vi "CRYSignal Path Table.vi"(11 "Calibration":T1[](array[typedef]) {"Sens Curve"."Z data" items=["dB", "Lin"]; "Sens Curve"."X data" items=["dB", "Lin"]; "Sens Curve"."Y data" items=["dB", "Lin"]; "Sens Curve"."Z dB ref" format="%.1f"; "Sens Curve"."Z axis" items=["Log", "Lin"]; "Sens Curve"."X dB ref" format="%.1f"; "Sens Curve"."X axis" items=["Log", "Lin"]; "Sens Curve"."Y axis" items=["Log", "Lin"]; "Sens Curve"."Y dB ref" format="%.1f"; "Sens Curve"."Curve"."z" format="%.2f"; "Sens Curve"."Curve"."y" format="%.2f"; "Sens Curve"."Curve"."x" format="%.2f"; "EQ Curve"."Z data" items=["dB", "Lin"]; "EQ Curve"."X data" items=["dB", "Lin"]; "EQ Curve"."Y data" items=["dB", "Lin"]; "EQ Curve"."Z dB ref" format="%.1f"; "EQ Curve"."Z axis" items=["Log", "Lin"]; "EQ Curve"."X dB ref" format="%.1f"; "EQ Curve"."X axis" items=["Log", "Lin"]; "EQ Curve"."Y axis" items=["Log", "Lin"]; "EQ Curve"."Y dB ref" format="%.1f"; "EQ Curve"."Curve"."z" format="%.2f"; "EQ Curve"."Curve"."y" format="%.2f"; "EQ Curve"."Curve"."x" format="%.2f"; "Corr Curve"."Z data" items=["dB", "Lin"]; "Corr Curve"."X data" items=["dB", "Lin"]; "Corr Curve"."Y data" items=["dB", "Lin"]; "Corr Curve"."Z dB ref" format="%.1f"; "Corr Curve"."Z axis" items=["Log", "Lin"]; "Corr Curve"."X dB ref" format="%.1f"; "Corr Curve"."X axis" items=["Log", "Lin"]; "Corr Curve"."Y axis" items=["Log", "Lin"]; "Corr Curve"."Y dB ref" format="%.1f"; "Corr Curve"."Curve"."z" format="%.2f"; "Corr Curve"."Curve"."y" format="%.2f"; "Corr Curve"."Curve"."x" format="%.2f"; "Calibration"."EQ Step size" items=["R10", "R20", "R40", "R80", "User"]; "Calibration"."Corr Step size" items=["R10", "R20", "R40", "R80", "User"]}) -> ()   [LabVIEW 2013]
uses:
  Typedef Control/CRYCalibration 2DCluster.ctl
  Typedef Control/CRYCalibration Cluster.ctl
  Typedef Control/CRYData Cluster.ctl
panel:
  out "OutputTable":string[][](table) caption="aaa"
  in  "OK":bool
  out "InputTable":string[][](table) caption="aaa"
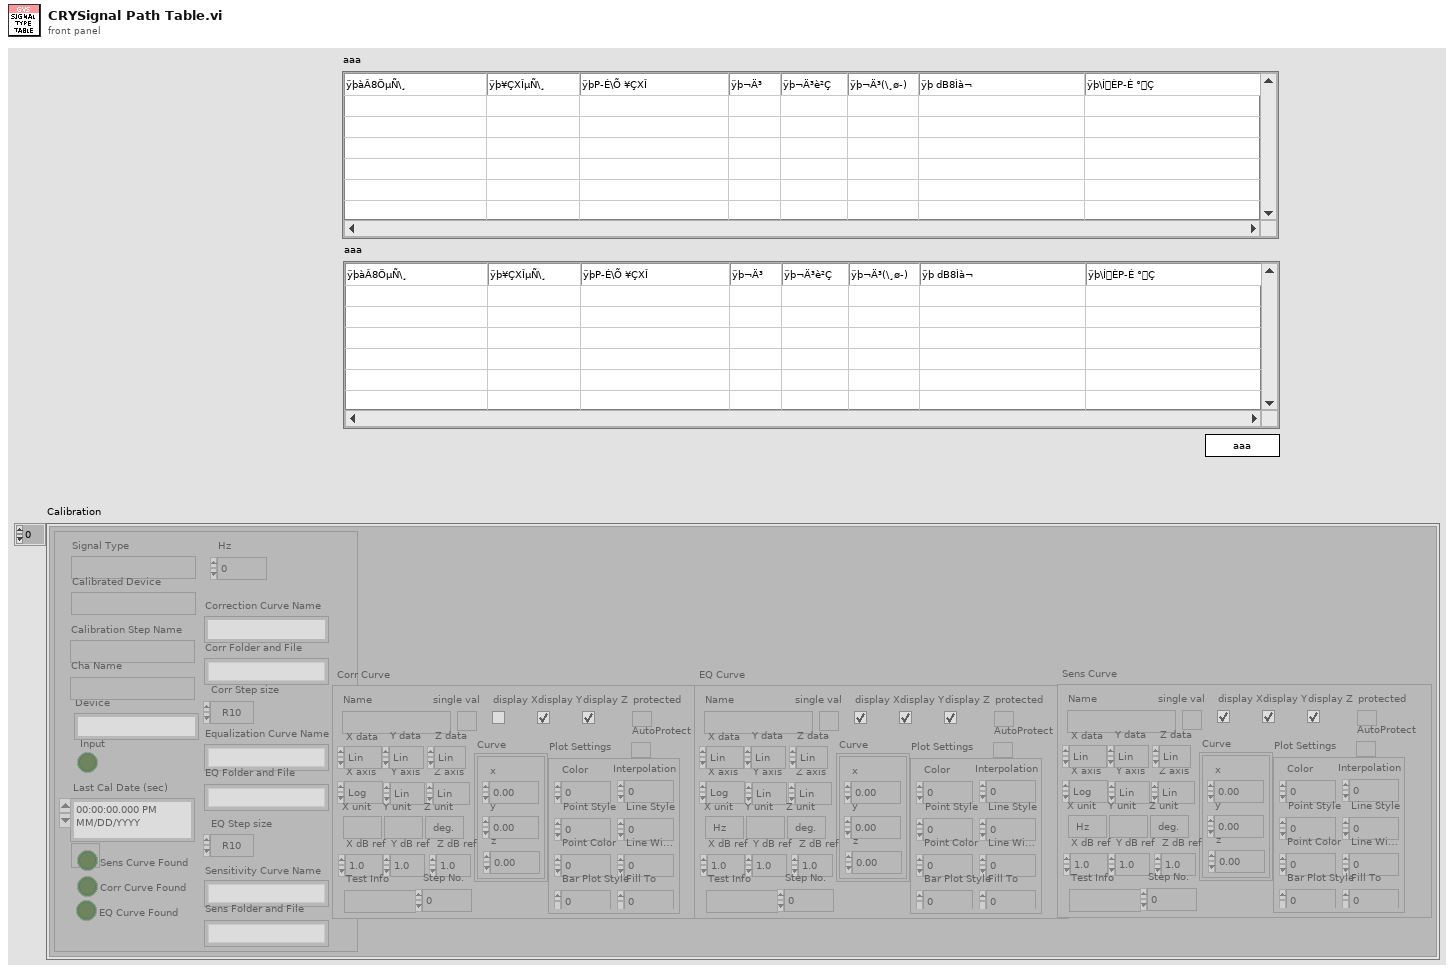
[diagram p1: front panel]
types:
  T1 = typedef "CRYCalibration 2DCluster.ctl" = cluster{"Calibration":T2, "Corr Curve":T3, "EQ Curve":T3, "Sens Curve":T3}
  T2 = typedef "CRYCalibration Cluster.ctl" = cluster{"Calibration Step Name":string, "Device":string, "Correction Curve Name":string, "Equalization Curve Name":string, "Sensitivity Curve Name":string, "Corr Folder and File":string, "EQ Folder and File":string, "Sens Folder and File":string, "Corr Step size":u16, "EQ Step size":u16, "Input":bool, "Last Cal Date (sec)":timestamp, "Cha Name":string, "Corr Curve Found":bool, "EQ Curve Found":bool, "Sens Curve Found":bool, "Signal Type":string, "Calibrated Device":string, "Hz":u32}
  T3 = typedef "CRYData Cluster.ctl" = cluster{"Name":string, "Curve":cluster{"x":dbl, "y":dbl, "z":dbl}[], "X data":u16, "Y data":u16, "Z data":u16, "X axis":u16, "Y axis":u16, "Z axis":u16, "X unit":string, "Y unit":string, "Z unit":string, "X dB ref":dbl, "Y dB ref":dbl, "Z dB ref":dbl, "single val":bool, "protected":bool, "display X":bool, "display Y":bool, "display Z":bool, "Test Info":string, "Step No.":i32, "Plot Settings":cluster{"Color":u32, "Interpolation":u8, "Point Style":u8, "Line Style":u8, "Point Color":u32, "Line Width":u8, "Bar Plot Style":u8, "Fill To":i16}, "AutoProtect":bool}
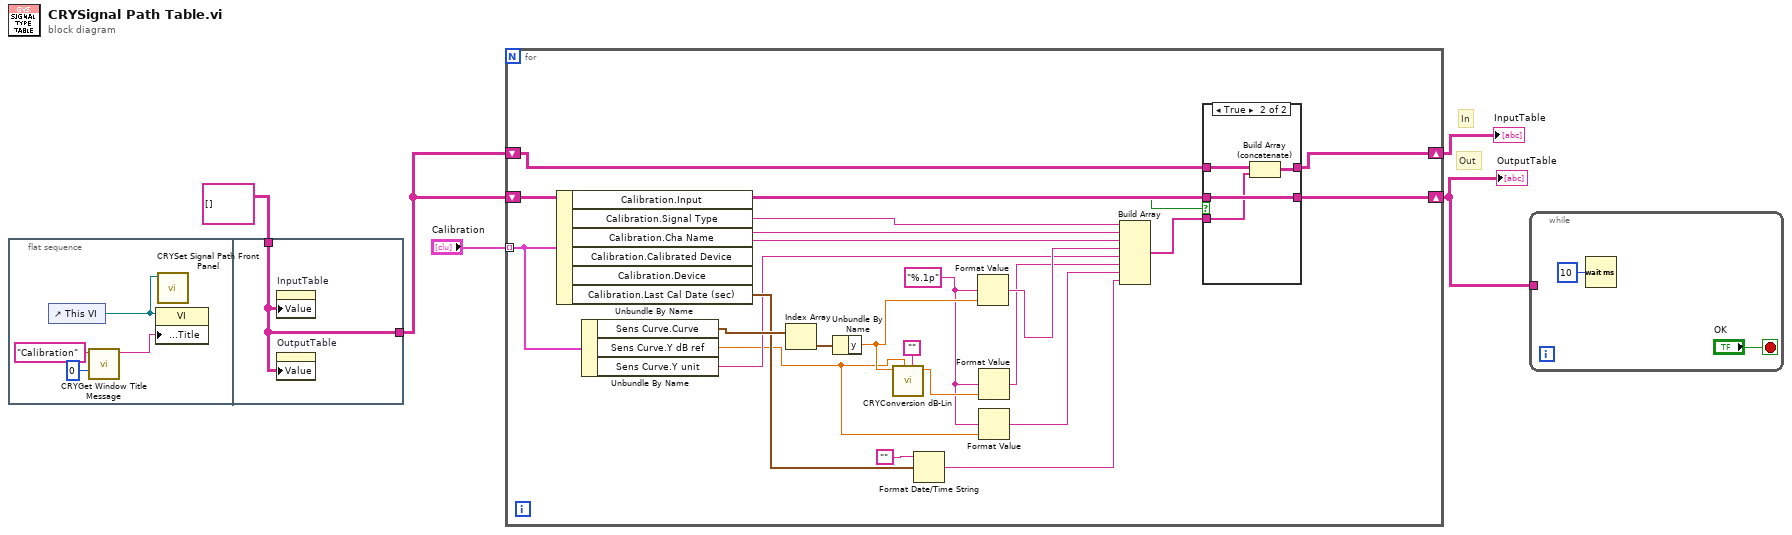
[diagram p0: block diagram]
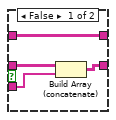
[diagram p2: hidden frame]
diagram:
  # "Out"
  # "In"
  n1 = flat-sequence {
    tunnel: string[][] [] ("Array") -> [w10]
    tunnel: [w10] -> w3
    frame #0 {
      n2 = control-ref of="This VI"() -> (w6:refnum<vi>)
      n3 = call "CRYGet Window Title Message.vi"("No"=0, "Kind"="Calibration") -> ("Multibyte String"=w7:string)  [unwired: 4 in, 5 out]
      n4 = property class="VI"(reference=w6, "Front Panel.Title"=w7) -> ()  [unwired: 1 in, 2 out]
      n5 = call "CRYSet Signal Path Front Panel.vi"("Vi Ref"=w6) -> ()  [unwired: 11 in]
    }
    frame #1 {
      n6 = property on="InputTable" class="Tbl (strict)"("Value"=w10) -> ()  [unwired: 2 in, 2 out]
      n7 = property on="OutputTable" class="Tbl (strict)"("Value"=w10) -> ()  [unwired: 2 in, 2 out]
    }
  }
  n8 = for {
    tunnel: "Calibration" -> [w28] mode=indexing
    shift-right: [w19] -> w2
    shift-left: w3 -> [w22]
    shift-right: [w18] -> w1
    shift-left: w3 -> [w21]
    w13 = "%.1p" ("format string")
    n9 = Unbundle By Name(w28) -> ("Calibration.Input"=w17:bool, "Calibration.Signal Type"=w27:string, "Calibration.Cha Name"=w26:string, "Calibration.Calibrated Device"=w25:string, "Calibration.Last Cal Date (sec)"=w23:timestamp)  [unwired: 1 out]
    n10 = Unbundle By Name(w28) -> ("Sens Curve.Curve"=w34:cluster{"x":dbl, "y":dbl, "z":dbl}[], "Sens Curve.Y dB ref"=w12:dbl, "Sens Curve.Y unit"=w15:string)
    n11 = Index Array(array=w34) -> (element=w33:cluster{"x":dbl, "y":dbl, "z":dbl})  [unwired: 1 in]
    n12 = Unbundle By Name(w33) -> ("y"=w30:dbl)
    n13 = call "CRYConversion dB-Lin.vi"("unit prefix"="", "dB ref."=w12, "Lin In"=w30) -> ("Log Out"=w29:dbl)  [unwired: 3 in, 3 out]
    n14 = Format Date/Time String(time format string (%c)="", seconds (now)=w23) -> (date/time string=w16:string)  [unwired: 1 out]
    n15 = Format Value(format string=w13, value (0)=w30) -> (output string=w24:string)  [unwired: 1 in]
    n16 = Format Value(format string=w13, value (0)=w29) -> (output string=w14:string)  [unwired: 1 in]
    n17 = Format Value(format string=w13, value (0)=w12) -> (output string=w11:string)  [unwired: 1 out]
    n18 = Build Array(w27, w26, w25, w24, w15, w14, w11, w16) -> (w20:string[])
    n19 = case shown="True" w17 {
      tunnel: w22 -> [w38 w41]
      tunnel: w21 -> [w37 w42]
      tunnel: [w35 w42] -> w18
      tunnel: [w38 w39] -> w19
      tunnel: w20 -> [w36 w40]
      frame False {
        n20 = Build Array (concatenate)(w37, w36) -> (w35:string[][])
      }
      frame True {
        n21 = Build Array (concatenate)(w41, w40) -> (w39:string[][])
      }
    }
  }
  "InputTable" <- w2
  "OutputTable" <- w1
  n22 = while {
    tunnel: w1 -> [_]
    stop <- "OK" stop-if-true
    n23 = Wait (ms)(milliseconds to wait=u32 10) -> ()  [unwired: 1 out]
  }
